vi "Clear Reservation.vi"(0 "object in":refnum<class "HPS-17000-PowerModule.lvclass">, 11 "Error In":errorcluster) -> (4 "object out":refnum<class "HPS-17000-PowerModule.lvclass">, 15 "Error Out":errorcluster)   [LabVIEW 2023, in "HPS-17000-PowerModule.lvlib" / "HPS-17000-PowerModule.lvclass"]
uses:
  HPS-17000-PowerModule.lvclass
  <instrlib>/HPS-17000/Internal/Clear Reservation Multi.vi
  <instrlib>/HPS-17000/Internal/Clear Reservation Confirmation Multi.vi
  <instrlib>/HPS-17000/HPS-17000.lvclass
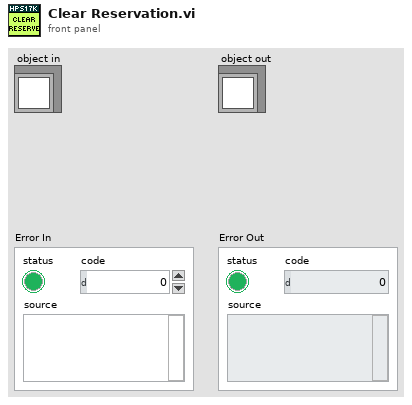
[diagram p1: front panel]
types:
  T1 = typedef "HPS-17000-PowerModule.lvlib/HPS-17000-PowerModule.lvclass/ObjectAttributes.ctl" = cluster{"HPS17000 IP Addresses":string[], "HPS Topology":enum16{"SINGLE", "MULTI"}, "GM ID":string, "TSN NIC IP Address":string, "HPS17000 Refs":refnum<class "HPS-17000.lvclass">[], "Stream Queues":refnum<queue>[], "connected":bool, "reserved":bool, "events":T2, "nibatterycycler_grpc_Setpoint":T3, "last timestamp":i64, "setpoint stream config":T4, "mode":T5, "range":T6}
  T2 = typedef "HPS-17000.lvclass/Multi-Cycler Events.ctl" = cluster{"heartbeats events":refnum<user-event>[], "faults events":refnum<user-event>[], "network sync event":refnum<user-event>[], "setpoint status event":refnum<user-event>[]}
  T3 = typedef "NI_BC_client.lvlib/nibatterycycler_grpc_Setpoint.ctl" = cluster{"voltage":sgl, "current":sgl, "min_power":sgl, "max_power":sgl, "resistance":sgl}
  T4 = typedef "Cycler.lvclass/Setpoint Stream Basic Config.ctl" = cluster{"local address":string, "receiver port":u16}
  T5 = typedef "HPS-17000-PowerModule.lvlib/HPS-17000-PowerModule.lvclass/Mode.ctl" = u16
  T6 = typedef "PowerModuleInterface.lvlibp/PowerModuleInterface.lvclass/Range.ctl" = cluster{"Current Max (A)":dbl, "Current Min (A)":dbl, "Voltage Max (V)":dbl, "Voltage Min (V)":dbl}
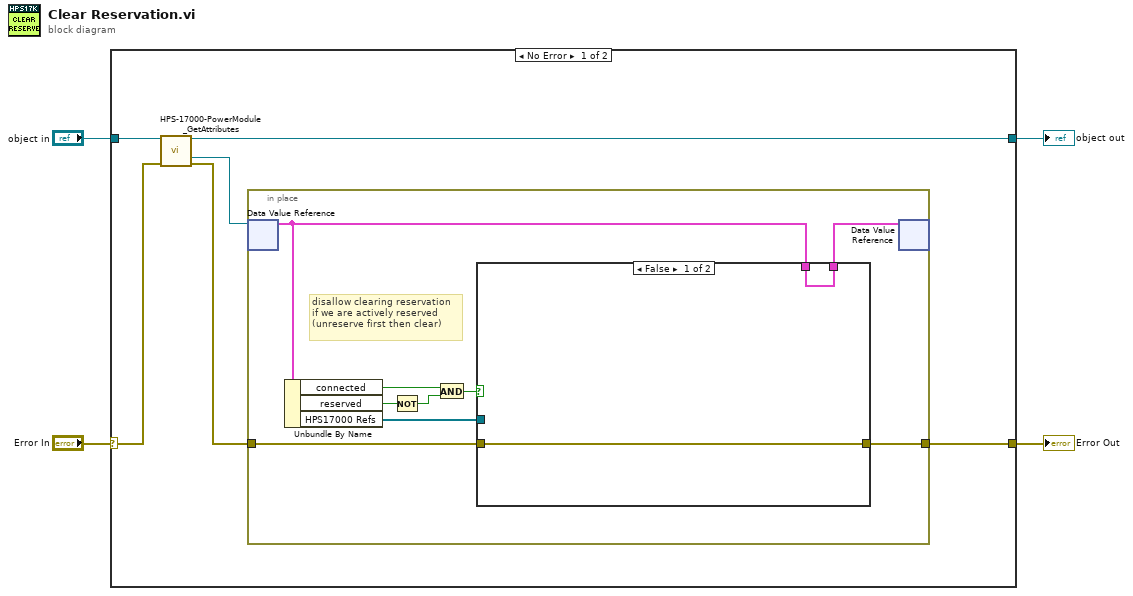
[diagram p0: block diagram]
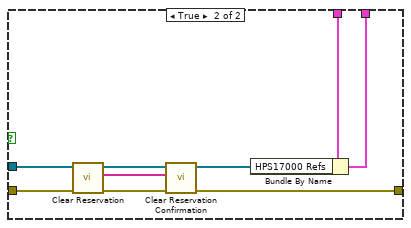
[diagram p2: hidden frame]
diagram:
  n1 = case shown="No Error" "Error In" {
    selector: "Error In" -> [w9 w31]
    tunnel: "object in" -> [w10 w32]
    tunnel: [w5 w32] -> w4
    tunnel: [w6 w31] -> w3
    frame No Error {
      n2 = call "HPS-17000-PowerModule_GetAttributes.vi"("reference in"=w10, "Error In"=w9) -> ("reference out"=w5:refnum<class "HPS-17000-PowerModule.lvclass">, "DataRef"=w8:refnum<data-value>, "Error Out"=w7:errorcluster)  [unwired: 10 in, 1 out]
      n3 = in-place {
        in-place-border: w7 -> [w17]
        in-place-border: [w16] -> w6
        # "disallow clearing reservation\nif we are actively reserved\n(unreserve first then clear)"
        n4 = in-place-dvr #1(w8) -> (w18:T1)  [unwired: 1 out]
        n5 = Unbundle By Name(w18) -> ("connected"=w14:bool, "reserved"=w12:bool, "HPS17000 Refs"=w15:refnum<class "HPS-17000.lvclass">[])
        n6 = Not(x=w12) -> (.not. x?=w11:bool)
        n7 = And(x=w14, y=w11) -> (x .and. y?=w13:bool)
        n8 = case shown="False" w13 {
          tunnel: [w21 w30] -> w19
          tunnel: w18 -> [w21 w29]
          tunnel: w17 -> [w20 w28]
          tunnel: [w20 w25] -> w16
          tunnel: w15 -> [_ w27]
          frame False {
          }
          frame True {
            n9 = call-poly <instrlib>:"Clear Reservation.vi"("error in"=w28, "cycler refs in"=w27) -> ("error out"=w26:errorcluster, "clear reserve tokens"=w22:string[], "cycler refs out"=w23:refnum<class "HPS-17000.lvclass">[])  [unwired: 7 in]
            n10 = call-poly <instrlib>:"Clear Reservation Confirmation.vi"("error in"=w26, "clear reserve tokens"=w22, "cycler refs in"=w23) -> ("error out"=w25:errorcluster, "cycler refs out"=w24:refnum<class "HPS-17000.lvclass">[])  [unwired: 7 in]
            n11 = Bundle By Name(cluster=w29, "HPS17000 Refs"=w24) -> (w30:T1)
          }
        }
        n12 = in-place-dvr #1(w19) -> ()  [unwired: 2 out]
      }
    }
    frame Error {
    }
  }
  "Error Out" <- w3
  "object out" <- w4
